vi "Realsense Cam Frame Store.vi"(4 "Width":i32, 5 "Depths":sgl[][](array[numeric]), 6 "Height":i32, 7 "Bytes":u8[](array[numeric]), 8 "error in (no error)":errorcluster, 9 "16-Bit IR":u16[](array[numeric]), 10 "Stream type":T1(ring), 11 "Realsense Cam in":refnum<class "Realsense Cam.lvclass">) -> (0 "error out":errorcluster, 3 "Realsense Cam out":refnum<class "Realsense Cam.lvclass">)   [LabVIEW 2018, in "Realsense Cam.lvclass"]
uses:
  Realsense Cam.lvclass
  Realsense Cam.lvclass/Realsense Cam.ctl
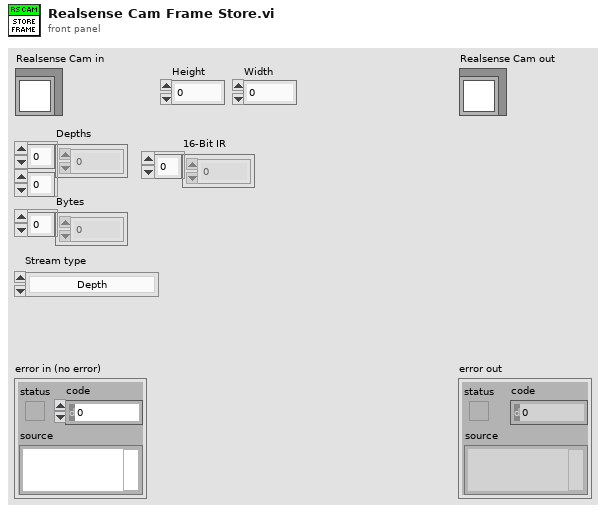
[diagram p1: front panel]
types:
  T1 = enum16{"Depth", "Color (ext.)", "Color (left) ", "IR Left", "IR Right", "IR Left (Y16)", "IR Right (Y16)"}
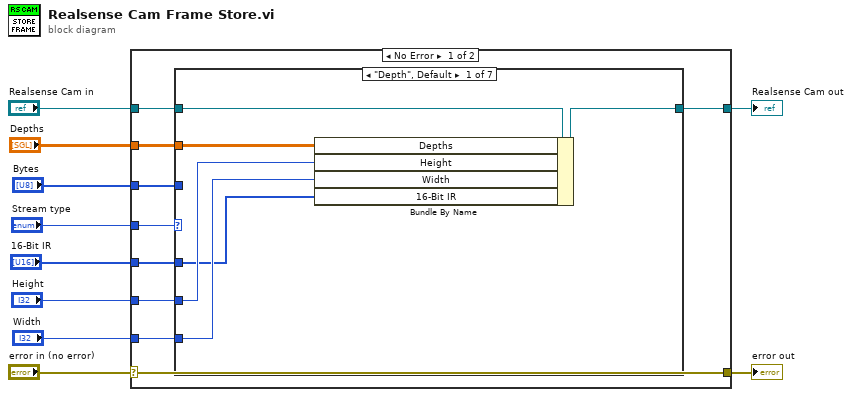
[diagram p0: block diagram]
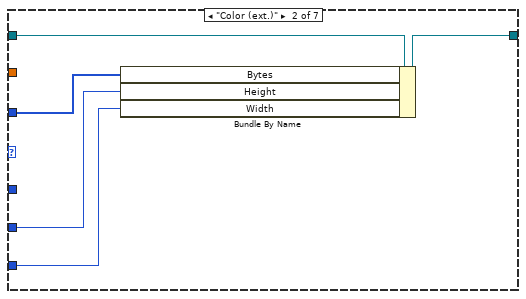
[diagram p2: hidden frame]
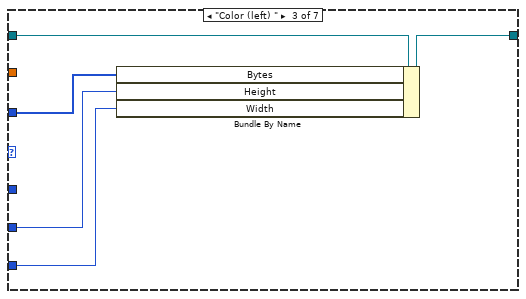
[diagram p3: hidden frame]
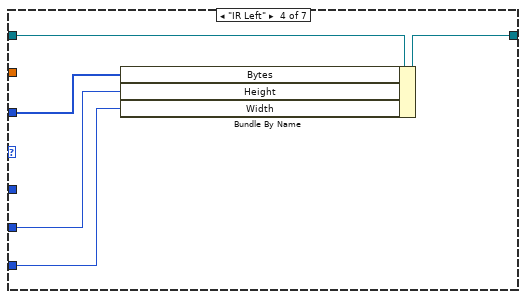
[diagram p4: hidden frame]
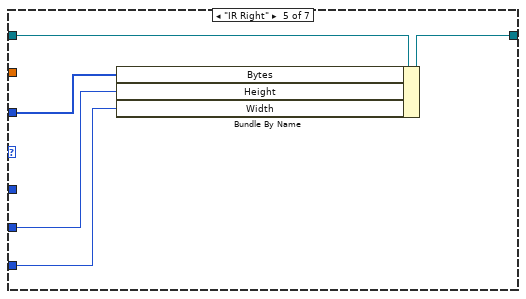
[diagram p5: hidden frame]
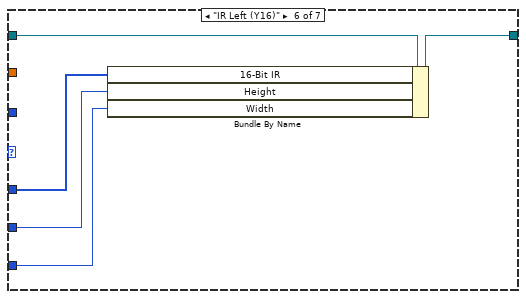
[diagram p6: hidden frame]
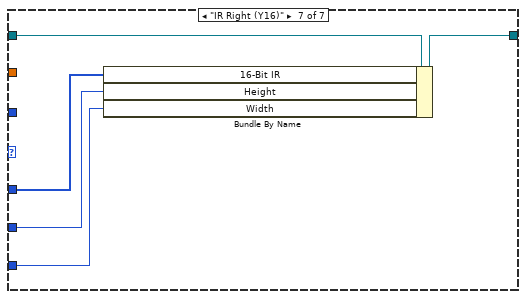
[diagram p7: hidden frame]
diagram:
  n1 = case shown="No Error" "error in (no error)" {
    selector: "error in (no error)" -> [w19 w57]
    tunnel: [w19 w57] -> w9
    tunnel: [w16 w56] -> w7
    tunnel: "Realsense Cam in" -> [w17 w56]
    tunnel: "Stream type" -> [w18 _]
    tunnel: "Depths" -> [w15 _]
    tunnel: "Bytes" -> [w14 _]
    tunnel: "Height" -> [w13 _]
    tunnel: "Width" -> [w12 _]
    tunnel: "16-Bit IR" -> [w11 _]
    frame No Error {
      n2 = case shown="\"Depth\", Default" w18 {
        tunnel: w17 -> [w25 w30 w35 w40 w45 w50 w55]
        tunnel: [w23 w28 w33 w38 w43 w49 w54] -> w16
        tunnel: w15 -> [w24 _ _ _ _ _ _]
        tunnel: w14 -> [_ w29 w34 w39 w44 _ _]
        tunnel: w13 -> [w22 w27 w32 w37 w42 w48 w53]
        tunnel: w12 -> [w21 w26 w31 w36 w41 w47 w52]
        tunnel: w11 -> [w20 _ _ _ _ w46 w51]
        frame "Depth", Default {
          n3 = Bundle By Name(cluster=w25, "Depths"=w24, "Height"=w22, "Width"=w21, "16-Bit IR"=w20) -> (w23:refnum<class "Realsense Cam.lvclass">)
        }
        frame "Color (ext.)" {
          n4 = Bundle By Name(cluster=w30, "Bytes"=w29, "Height"=w27, "Width"=w26) -> (w28:refnum<class "Realsense Cam.lvclass">)
        }
        frame "Color (left) " {
          n5 = Bundle By Name(cluster=w35, "Bytes"=w34, "Height"=w32, "Width"=w31) -> (w33:refnum<class "Realsense Cam.lvclass">)
        }
        frame "IR Left" {
          n6 = Bundle By Name(cluster=w40, "Bytes"=w39, "Height"=w37, "Width"=w36) -> (w38:refnum<class "Realsense Cam.lvclass">)
        }
        frame "IR Right" {
          n7 = Bundle By Name(cluster=w45, "Bytes"=w44, "Height"=w42, "Width"=w41) -> (w43:refnum<class "Realsense Cam.lvclass">)
        }
        frame "IR Left (Y16)" {
          n8 = Bundle By Name(cluster=w50, "16-Bit IR"=w46, "Height"=w48, "Width"=w47) -> (w49:refnum<class "Realsense Cam.lvclass">)
        }
        frame "IR Right (Y16)" {
          n9 = Bundle By Name(cluster=w55, "16-Bit IR"=w51, "Height"=w53, "Width"=w52) -> (w54:refnum<class "Realsense Cam.lvclass">)
        }
      }
    }
    frame Error {
    }
  }
  "error out" <- w9
  "Realsense Cam out" <- w7
